vi "FFT half.vi"(1 "X[1..N]":i32[](array[numeric])) -> (0 "FFT(X)[1..N/2]":dbl[](array[numeric]) format="%.2f")   [LabVIEW 2009]
uses:
  <vilib>/Analysis/2dsp.llb/Real FFT.vi
  <vilib>/Analysis/NI_AALPro.lvlib
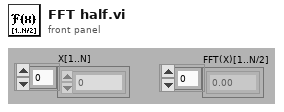
[diagram p1: front panel]
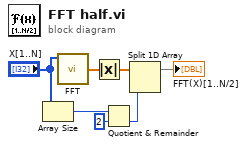
[diagram p0: block diagram]
diagram:
  n1 = Array Size(array="X[1..N]") -> (size(s)=w7:i32)
  n2 = call-poly <vilib>:"FFT.vi"("X"="X[1..N]") -> ("FFT {X}"=w3:cdb[])  [unwired: 9 in, 1 out]
  n3 = Absolute Value(x=w3) -> (abs(x)=w4:dbl[])
  n4 = Quotient & Remainder(x=w7, y=2) -> (floor(x/y)=w5:i32)  [unwired: 1 out]
  n5 = Split 1D Array(array=w4, index=w5) -> (first subarray=→"FFT(X)[1..N/2]":dbl[])  [unwired: 1 out]
